vi "Pressurise.vi"(8 "error in (no error)":errorcluster, 9 "Measuring Limb":string, 10 "SignalCluster in":T1, 11 "Queue in":refnum<queue>) -> (0 "error out":errorcluster, 3 "SignalCluster out":T1)   [LabVIEW 2013, in "main.lvlib"]
uses:
  main.lvlib
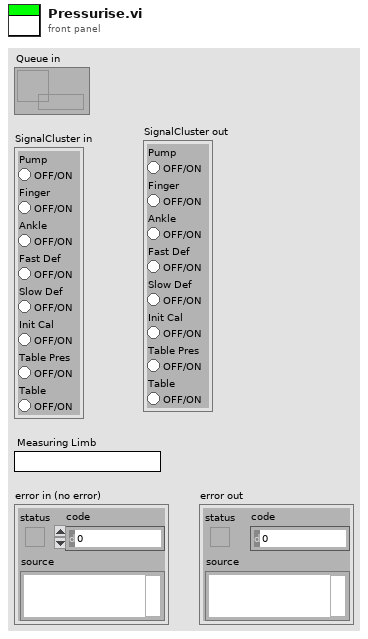
[diagram p1: front panel]
types:
  T1 = cluster{"Pump":bool, "Finger":bool, "Ankle":bool, "Fast Def":bool, "Slow Def":bool, "Init Cal":bool, "Table Pres":bool, "Table":bool}
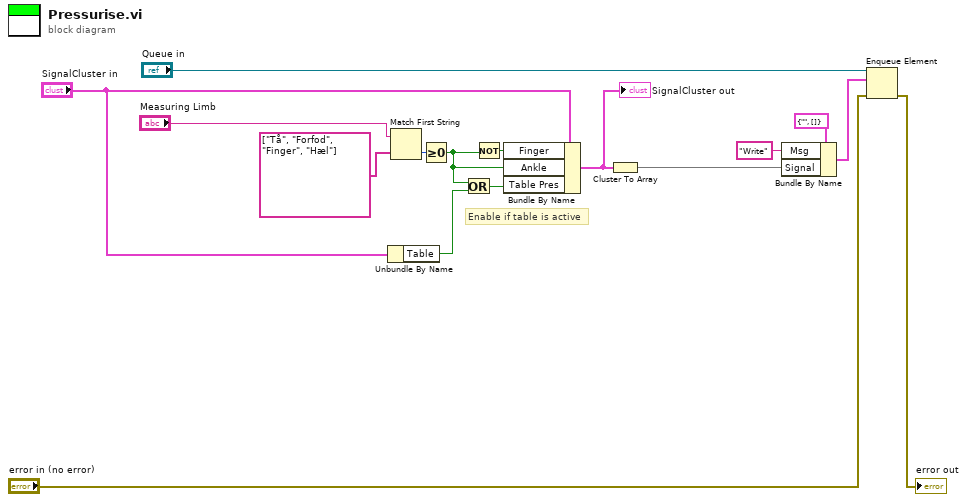
[diagram p0: block diagram]
diagram:
  # "Enable if table is active"
  n1 = Unbundle By Name("SignalCluster in") -> ("Table"=w16:bool)
  n2 = Match First String(2:string[] ["Tå", "Forfod", "Finger", "Hæl"], 3:"Measuring Limb") -> (0:w9:i32)  [unwired: 1 out]
  n3 = Greater Or Equal To 0?(x=w9) -> (x >= 0?=w15:bool)
  n4 = Or(x=w15, y=w16) -> (x .or. y?=w14:bool)
  n5 = Not(x=w15) -> (.not. x?=w10:bool)
  n6 = Bundle By Name(cluster="SignalCluster in", "Finger"=w10, "Ankle"=w15, "Table Pres"=w14) -> (w12:T1)
  "SignalCluster out" <- w12
  n7 = Cluster To Array(cluster=w12) -> (array=w11:bool[])
  n8 = Bundle By Name(cluster=cluster{"Msg":string, "Signal":bool[]} {"Msg"="", "Signal"=[]} ("element"), "Msg"="Write", "Signal"=w11) -> (w5:cluster{"Msg":string, "Signal":bool[]})
  n9 = Enqueue Element(queue="Queue in", element=w5, error in (no error)="error in (no error)") -> (error out=→"error out":errorcluster)  [unwired: 1 in, 2 out]
